vi "mag-field_set_B-field.vi"(10 "Field (T)":dbl min=0.0 max=16.0, 11 "GPIB adr in":string) -> (3 "GPIB adr out":string)   [LabVIEW 2010]
doc: "Sets the coil filed (assuming 120A mode on power supply).\nGive B value as positive number, and set the sign via the polarity\nconnector (true = plus sign)."
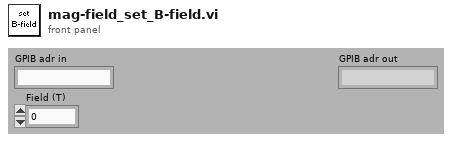
[diagram p1: front panel]
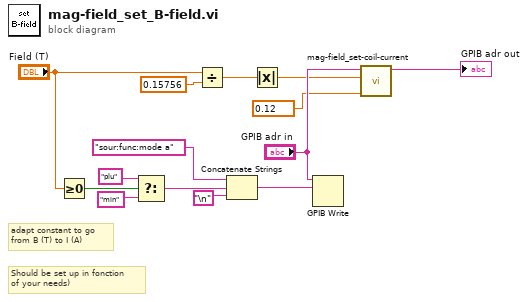
[diagram p0: block diagram]
diagram:
  w10 = 0.12 items=["12A"=0.012, "120A"=0.12] ("mode")
  # "adapt constant to go\nfrom B (T) to I (A)"
  # "Should be set up in fonction\nof your needs)"
  n1 = Greater Or Equal To 0?(x="Field (T)") -> (x >= 0?=w1:bool)
  n2 = Select(t="plu" ("GPIB adr in"), s=w1, f="min" ("GPIB adr in")) -> (s? t:f=w6:string)
  n3 = Divide(x="Field (T)", y=0.15756) -> (x/y=w12:dbl)
  n4 = Concatenate Strings("sour:func:mode a" ("string"), w6, "\n") -> (w3:string)
  n5 = Absolute Value(x=w12) -> (abs(x)=w9:dbl)
  n6 = GPIB Write(0:"GPIB adr in", 1:w3) -> ()  [unwired: 1 in, 4 out]
  n7 = call "mag-field_set-coil-current.vi"("mode"=w10, "Current (A)"=w9, "GPIB adr in"="GPIB adr in") -> ("GPIB adr out"=→"GPIB adr out":string)  [unwired: 8 out]
